vi "Frames to Channels.vi"(8 "error in (no error)":errorcluster, 9 "channel classification":T1, 10 "Frames":refnum<k21>[](array[refnum])) -> (0 "error out":errorcluster, 2 "Mappings out":T2[](array[typedef]))   [LabVIEW 2017, in "J1939 editor node.lvclass"]
uses:
  J1939 editor node.lvclass
  Mappings.ctl
  <vilib>/NI/Tag Bus Module Framework/channel/TBM channel.lvclass
  module/configuration/Line.ctl
  Map.ctl
  <vilib>/NI/Tag Bus Module Framework/channel/channel classification.ctl
  module/configuration/J1939 configuration.lvclass
  <resource>/objmgr/xnet.rc
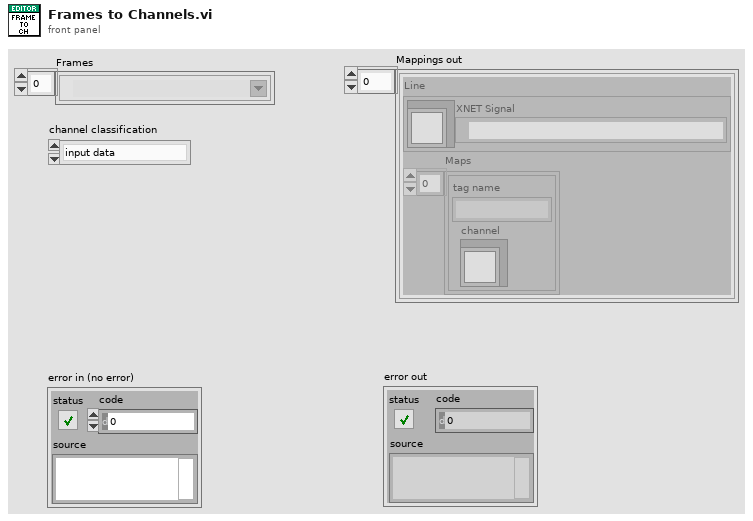
[diagram p1: front panel]
types:
  T1 = typedef "TBM channel.lvclass/channel classification.ctl" = enum16{"input data", "output data", "processing parameter", "processing result"}
  T2 = typedef "J1939 editor node.lvclass/Mappings.ctl" = cluster{"Line":T3, "Maps":T4[]}
  T3 = typedef "J1939 configuration.lvclass/Line.ctl" = cluster{"channel":refnum<class "TBM channel.lvclass">, "XNET Signal":refnum<k21>}
  T4 = typedef "J1939 editor node.lvclass/Map.ctl" = cluster{"channel":refnum<class "TBM channel.lvclass">, "tag name":string}
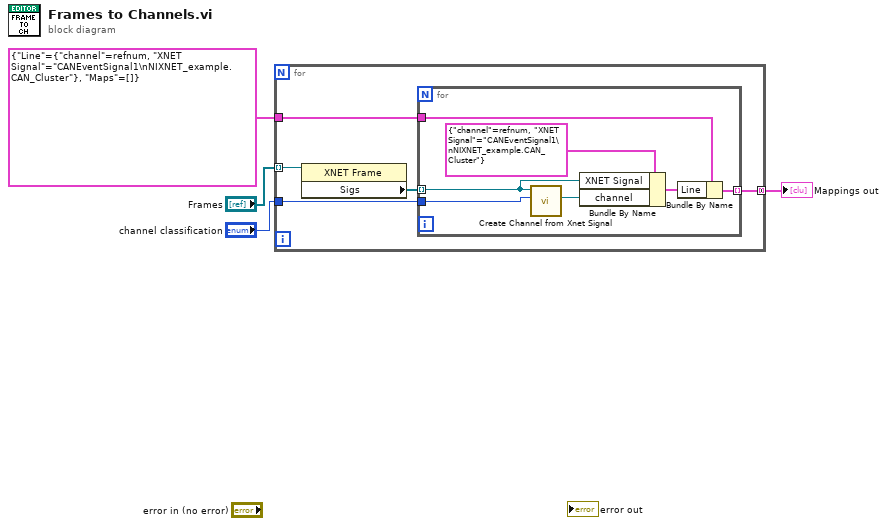
[diagram p0: block diagram]
diagram:
  n1 = for {
    tunnel: [w5] -> w4 mode=concatenating
    tunnel: T2 {"Line"={"channel"=refnum, "XNET Signal"="CANEventSignal1\nNIXNET_example.CAN_Cluster"}, "Maps"=[]} ("Mappings out") -> [w6]
    tunnel: "Frames" -> [w9] mode=indexing
    tunnel: "channel classification" -> [w7]
    n2 = property class="XNET Frame"(reference=w9) -> ("Sigs"=w8:refnum<k21>[])  [unwired: 1 in, 2 out]
    n3 = for {
      tunnel: w8 -> [w15] mode=indexing
      tunnel: w7 -> [w14]
      tunnel: w6 -> [w12]
      tunnel: [w10] -> w5 mode=indexing
      n4 = call "Create Channel from Xnet Signal.vi"("channel classification"=w14, "XNET Signal in"=w15) -> ("channel"=w13:refnum<class "TBM channel.lvclass">)  [unwired: 7 in, 2 out]
      n5 = Bundle By Name(cluster=T3 {"channel"=refnum, "XNET Signal"="CANEventSignal1\nNIXNET_example.CAN_Cluster"} ("Line"), "XNET Signal"=w15, "channel"=w13) -> (w11:T3)
      n6 = Bundle By Name(cluster=w12, "Line"=w11) -> (w10:T2)
    }
  }
  "Mappings out" <- w4
